vi "ief_get_send_flag.vi"(0 "tag prefix in":refnum<k21>, 1 "error in (no error)":errorcluster) -> (2 "Send-Flag":bool, 3 "value status":i32, 4 "error out (no error)":errorcluster)   [LabVIEW 2015, in "IEF Werner.lvlib"]
doc: "Gets the actual value of the command flag. This is necessary since the command flag has to be toggled before a command is executed."
uses:
  IEF Werner.lvlib
  Packages/CSPP_Core/Libraries/Base/FGV Action.ctl
  <vilib>/lvdsc/legacy/tag/legacy_Read_Tag_(analog)7x.vi
  Packages/CSPP_Core/Libraries/Base/CS++Base.lvlib
panel:
  out "First Time":bool=TRUE
  # "IEF Get Send Flag"
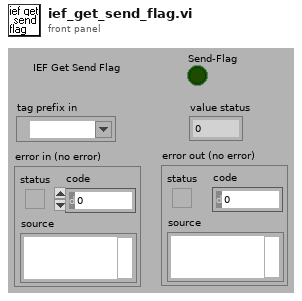
[diagram p1: front panel]
types:
  T1 = typedef "CS++Base.lvlib/FGV Action.ctl" = enum16{"add", "replace", "read", "remove", "reset", "get attributes"}
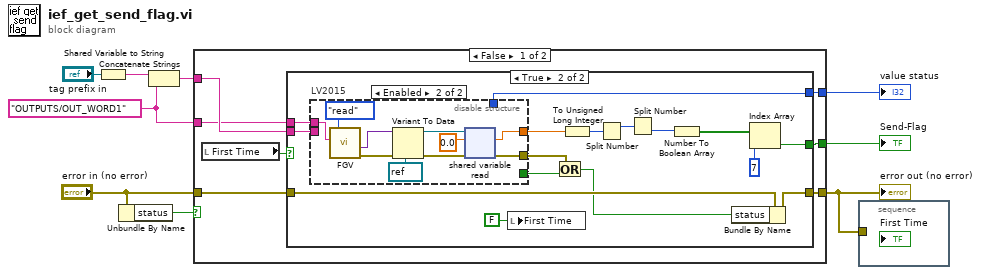
[diagram p0: block diagram]
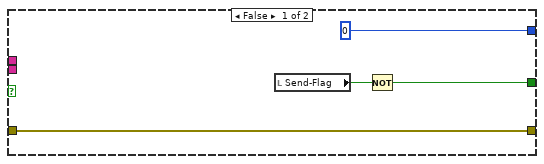
[diagram p2: hidden frame]
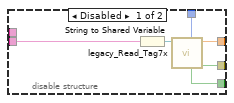
[diagram p3: hidden frame]
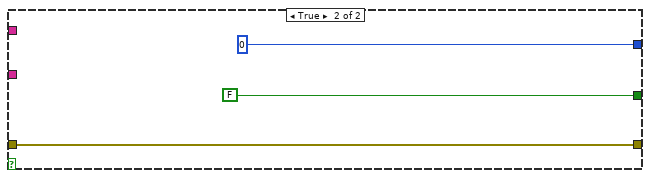
[diagram p4: hidden frame]
diagram:
  w1 = "OUTPUTS/OUT_WORD1"
  n1 = Shared Variable to String(1:"tag prefix in") -> (0:w5:string)
  n2 = Unbundle By Name("error in (no error)") -> ("status"=w6:bool)
  n3 = Concatenate Strings(w5, w1) -> (w3:string)
  n4 = case shown="False" w6 {
    tunnel: [w16 FALSE] -> w9
    tunnel: [w15 0 ("value status")] -> w8
    tunnel: [w12 w55] -> w2
    tunnel: "error in (no error)" -> [w13 w55]
    tunnel: w3 -> [w11 _]
    tunnel: w1 -> [w10 _]
    frame False {
      n5 = local read "First Time"() -> (w14:bool)
      n6 = case shown="True" w14 {
        tunnel: [w18 w33] -> w16
        tunnel: [0 ("value status") w32] -> w15
        tunnel: w13 -> [w17 w27]
        tunnel: [w17 w28] -> w12
        tunnel: w11 -> [_ w22]
        tunnel: w10 -> [_ w21]
        frame False {
          n7 = local read "Send-Flag"() -> (w19:bool)
          n8 = Not(x=w19) -> (.not. x?=w18:bool)
        }
        frame True {
          n9 = disable-structure "LV2015" shown="Enabled" {
            disable-tunnel: [w42 w51] -> w36
            disable-tunnel: [w41 _] -> w32
            disable-tunnel: [w40 w50] -> w31
            disable-tunnel: [w39 _] -> w30
            disable-tunnel: w22 -> [w38 _]
            disable-tunnel: w21 -> [_ w44]
            frame Disabled {
              n10 = String to Shared Variable(0:w38) -> (2:w37:refnum<k21>)  [unwired: 1 out]
              n11 = call-poly <vilib>:"legacy_Read_Tag7x.vi"("tag name"=w37) -> ("error"=w40:bool, "value"=w42:dbl, "shutdown"=w39:bool, "value status"=w41:i32)  [unwired: 4 in, 3 out]
            }
            frame Enabled {
              n12 = call "FGV.vi"("Attribute Name"=w44, "Action (read)"=FGV_Action."read") -> ("Error Out"=w49:errorcluster, "Data out"=w45:variant)  [unwired: 5 in, 3 out]
              n13 = Variant To Data(error in=w49, type=refnum<k21> refnum ("shared variable refnum in"), Variant=w45) -> (data=w46:refnum<k21>, error out=w48:errorcluster)
              n14 = shared-variable-read(w46, w48, 0.0) -> (w50:errorcluster, w51:dbl)  [unwired: 2 out]
            }
          }
          n15 = local write "First Time"(FALSE ("First Time")) -> ()
          n16 = Or(x=w31, y=w30) -> (x .or. y?=w26:bool)
          n17 = To Unsigned Long Integer(number=w36) -> (unsigned 32bit integer=w25:u32)
          n18 = Split Number(x=w25) -> (hi(x)=w24:u16)  [unwired: 1 out]
          n19 = Split Number(x=w24) -> (lo(x)=w23:u8)  [unwired: 1 out]
          n20 = Number To Boolean Array(number=w23) -> (Boolean array=w35:bool[])
          n21 = Bundle By Name(cluster=w27, "status"=w26) -> (w28:errorcluster)
          n22 = Index Array(array=w35, index=7 ("Index")) -> (element=w33:bool)
        }
      }
    }
    frame True {
    }
  }
  "Send-Flag" <- w9
  "value status" <- w8
  "error out (no error)" <- w2
  n23 = stacked-sequence {
    tunnel: w2 -> [_]
    frame #0 {
    }
  }
